vi "TDMS Properties.vi"() -> ()   [LabVIEW 2015]
uses:
  <vilib>/Utility/VariantDataType/Type.ctl
  <vilib>/measure/NI_MABase.lvlib
  <vilib>/Utility/VariantDataType/VariantType.lvlib
panel:
  in  "Group Name in":string
  in  "Channel Name in":string
  in  "file path":path
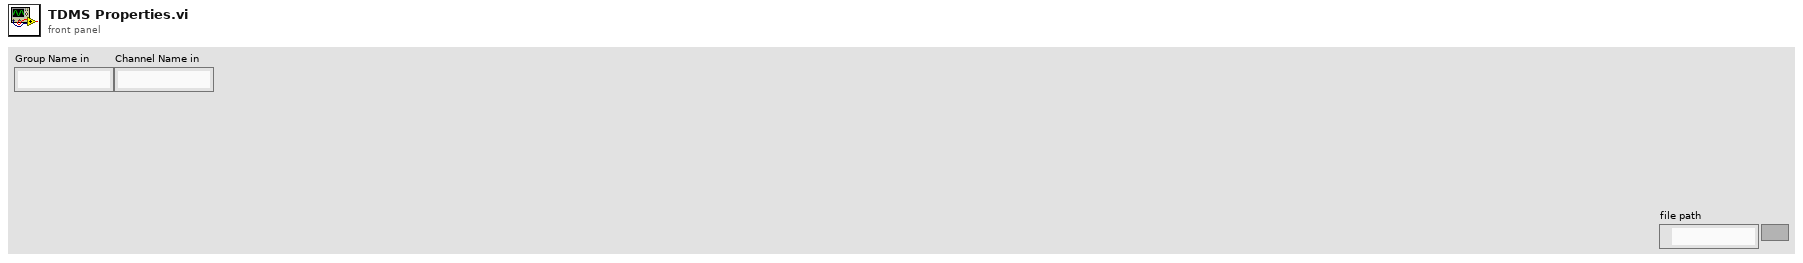
[diagram p1: front panel]
types:
  T1 = typedef "VariantType.lvlib/Type.ctl" = enum8{"Invalid Type", "Void", "I8", "I16", "I32", "I64", "U8", "U16", "U32", "U64", "Single Float", "Double Float", "Extended Float", "Single Complex", "Double Complex", "Extended Complex", "Enum U8", "Enum U16", "Enum U32", "Enum U64", "Single Float With Unit", "Double Float With Unit", "Extended Float With Unit", "Single Complex with Unit", "Double Complex with Unit", "Extended Complex with Unit", "Boolean", "String", "Path", "Picture", "Tag", "Array", "Cluster", "Variant", "LV Variant", "Waveform", "Timestamp", "Digital Waveform", "Digital Data", "ExpressData", "Refnum", "External Data", "VI", "Poly VI", "LabVIEW Class Instance", "Fixed Point"}
  T2 = enum16{"open", "open or create", "create or replace", "create", "open (read-only)"}
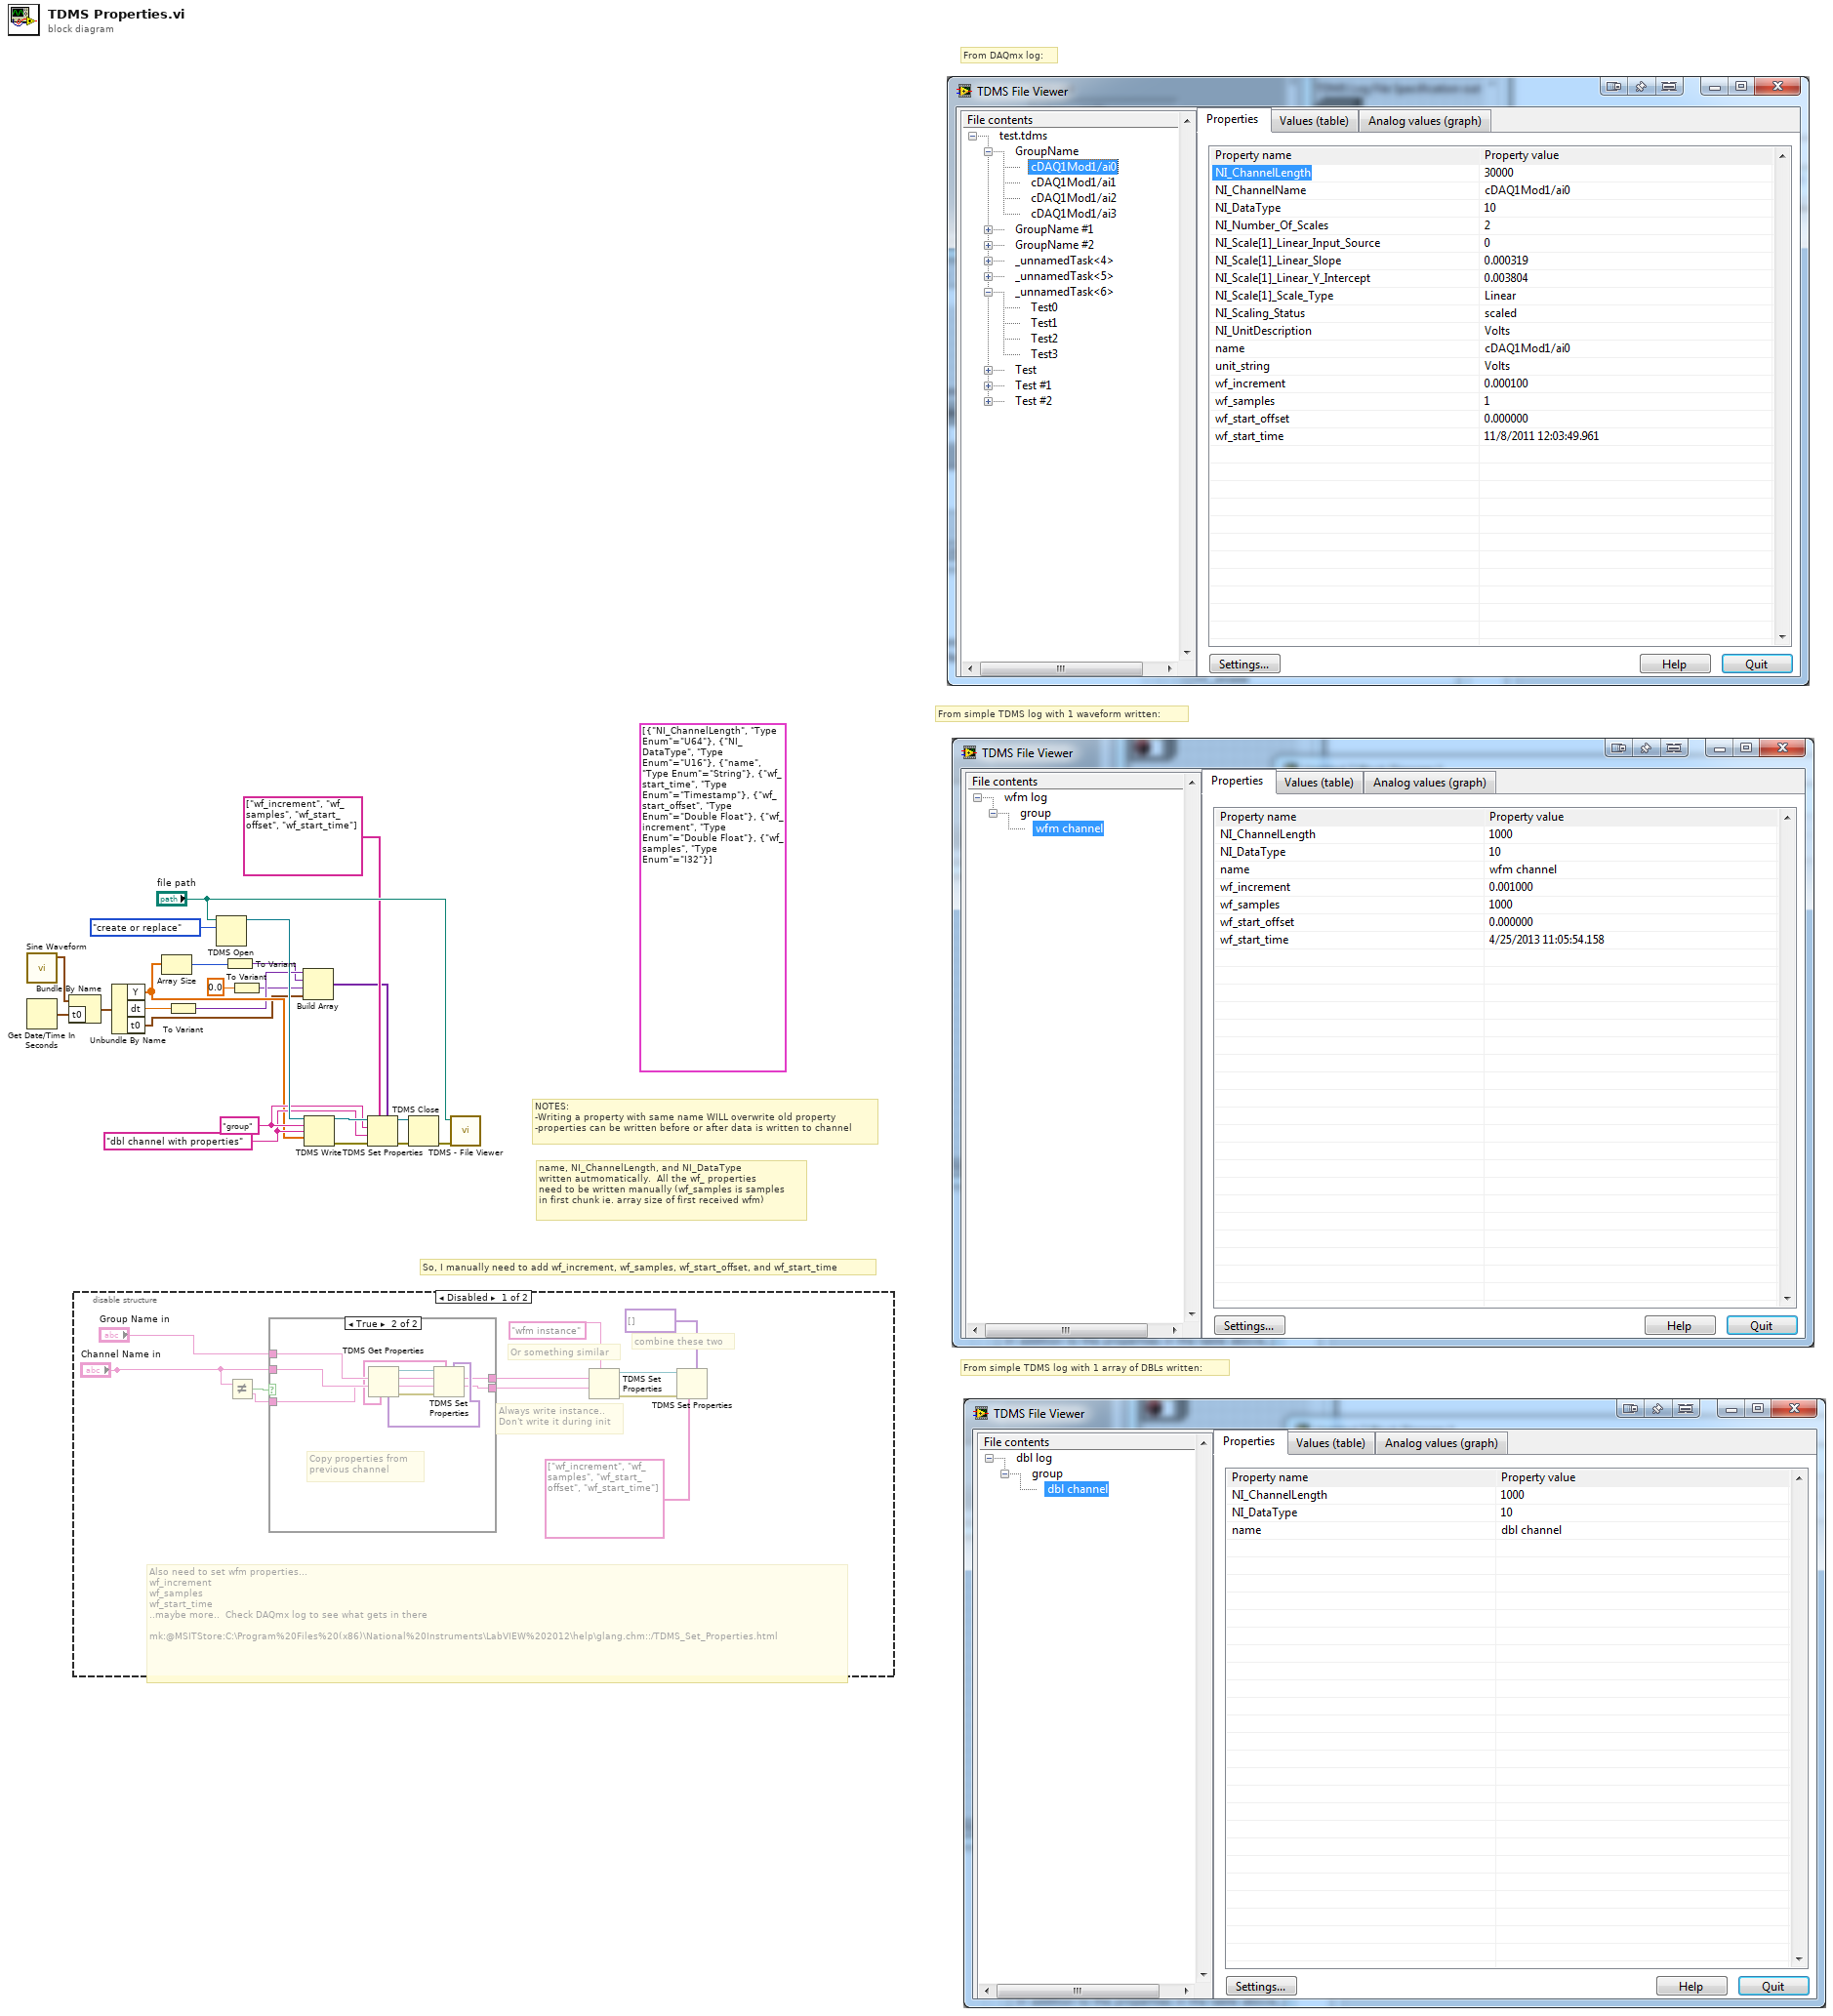
[diagram p0: block diagram]
diagram:
  (unwired) cluster{string, "Type Enum":T1}[] [{"NI_ChannelLength", "Type Enum"=enum."U64"}, {"NI_DataType", "Type Enum"=enum."U16"}, {"name", "Type Enum"=enum."String"}, {"wf_start_time", "Type Enum"=enum."Timestamp"}, {"wf_start_offset", "Type Enum"=enum."Double Float"}, {"wf_increment", "Type Enum"=enum."Double Float"}, {"wf_samples", "Type Enum"=enum."I32"}] ("Array 2")
  w14 = "dbl channel with properties" ("channel name(s) in (Untitled)")
  w15 = "group" ("group name in (Untitled)")
  # "From DAQmx log:"
  # "From simple TDMS log with 1 waveform written:"
  # "From simple TDMS log with 1 array of DBLs written:"
  # "So, I manually need to add wf_increment, wf_samples, wf_start_offset, and wf_start_time"
  # "name, NI_ChannelLength, and NI_DataType\nwritten autmomatically.  All the wf_ properties\nneed to be written manually (wf_samples is samples\nin first chunk ie. array size of first received wfm)"
  # "NOTES:\n-Writing a property with same name WILL overwrite old property\n-properties can be written before or after data is written to channel"
  n1 = call <vilib>:"Sine Waveform.vi"() -> ("signal out"=w13:waveform(dbl))  [unwired: 10 in, 1 out]
  n2 = Get Date/Time In Seconds() -> (seconds since 1Jan1904=w12:timestamp)
  n3 = Bundle By Name(cluster=w13, "t0"=w12) -> (w1:waveform(dbl))
  n4 = disable-structure shown="Disabled" {
    frame Disabled {
      # "Always write instance..\nDon't write it during init"
      # "combine these two"
      # "Or something similar"
      # "Also need to set wfm properties...\nwf_increment\nwf_samples\nwf_start_time\n..maybe more..  Check DAQmx log to see what gets in there\n\nmk:@MSITStore:C:\\Program%20Files%20(x86)\\National%20Instruments\\LabVIEW%202012\\help\\glang.chm::/TDMS_Set_Properties.html"
      n5 = Not Equal?(x="Channel Name in", y=w33) -> (x != y?=w32:bool)
      n6 = case shown="True" w32 {
        tunnel: "Group Name in" -> [_ w42]
        tunnel: "Channel Name in" -> [_ w41]
        tunnel: [_ w40] -> w33
        tunnel: [_ w37] -> w31
        tunnel: [_ w36] -> w30
        frame False {
        }
        frame True {
          # "Copy properties from \nprevious channel"
          n7 = TDMS Get Properties(9:w41, 10:w42) -> (0:w44:errorcluster, 2:w45:string, 3:w43:refnum<k34>, 4:w38:variant[], 6:w39:string[])  [unwired: 4 in, 1 out]
          n8 = TDMS Set Properties(5:w38, 7:w39, 8:w44, 9:w40, 10:w45, 11:w43) -> (1:w36:string, 2:w37:string)  [unwired: 2 out]
        }
      }
      n9 = TDMS Set Properties(7:"wfm instance" ("property names"), 9:w30, 10:w31) -> (0:w26:errorcluster, 3:w27:refnum<k34>, 5:w29:variant[])  [unwired: 2 in, 2 out]
      n10 = TDMS Set Properties(5:variant[] [] ("property values"), 7:string[] ["wf_increment", "wf_samples", "wf_start_offset", "wf_start_time"] ("property names"), 8:w26, 11:w27) -> ()  [unwired: 2 in, 4 out]
    }
    frame Enabled {
    }
  }
  n11 = Unbundle By Name(w1) -> ("Y"=w10:dbl[], "dt"=w9:dbl, "t0"=w3:timestamp)
  n12 = Array Size(array=w10) -> (size(s)=w6:i32)
  n13 = To Variant(anything=w9) -> (Variant=w8:variant)
  n14 = TDMS Open(10:T2."create or replace" ("operation (0:open)"), 11:"file path") -> (3:w22:refnum<k34>)  [unwired: 5 in, 1 out]
  n15 = To Variant(anything=w6) -> (Variant=w7:variant)
  n16 = To Variant(anything=0.0) -> (Variant=w4:variant)
  n17 = Build Array(w8, w7, w4, w3) -> (w2:variant[])
  n18 = TDMS Write(0:w22, 5:w15, 7:w14, 9:w10) -> (4:w18:refnum<k34>, 15:w19:errorcluster)  [unwired: 2 in, 2 out]
  n19 = TDMS Set Properties(5:w2, 7:string[] ["wf_increment", "wf_samples", "wf_start_offset", "wf_start_time"] ("property names"), 8:w19, 9:w14, 10:w15, 11:w18) -> (0:w16:errorcluster, 3:w17:refnum<k34>)  [unwired: 2 out]
  n20 = TDMS Close(8:w16, 11:w17) -> (0:w21:errorcluster)  [unwired: 1 out]
  n21 = call <vilib>:"TDMS - File Viewer.vi"("error in (no error)"=w21, "file path"="file path") -> ()  [unwired: 4 in, 2 out]
